vi "FourBarBoth.vi"(10 "Down":dbl, 11 "Up":dbl) -> ()   [LabVIEW 2018]
uses:
  <vilib>/Rock Robotics/WPI/ThirdParty/Phoenix-LabVIEW/Motor Controller/Controls/CTRE_Phoenix_MotorControl_ControlMode.ctl
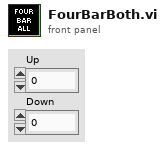
[diagram p1: front panel]
types:
  T1 = typedef "WPI_DigitalInputDevRef.ctl" = cluster{"DevStatus":errorcluster, "DIO Channel":T2}
  T2 = typedef "FPGA_DIOChannel.ctl" = enum8{"DIO 0", "DIO 1", "DIO 2", "DIO 3", "DIO 4", "DIO 5", "DIO 6", "DIO 7", "DIO 8", "DIO 9", "DIO MXP 0", "DIO MXP 1", "DIO MXP 2", "DIO MXP 3", "DIO MXP 4", "DIO MXP 5", "DIO MXP 6", "DIO MXP 7", "DIO MXP 8", "DIO MXP 9", "DIO MXP 10", "DIO MXP 11", "DIO MXP 12", "DIO MXP 13", "DIO MXP 14", "DIO MXP 15", "SPI Port CS1", "SPI Port CS2", "SPI Port CS3", "SPI Port MISO", "SPI Port MOSI", "Invalid"}
  T3 = typedef "CTRE_Phoenix_MotorControl_ControlMode.ctl" = u16
  T4 = typedef "WPI_MotorControlDeviceRef.ctl" = cluster{"DeviceStatus":errorcluster, "Type":T5, "PWM":cluster{"PWM Channel":T6, "DeadBand":T7}, "CAN":cluster{"Device Number":u8, "SetOutput VI Ref":variant, "GetOutput VI Ref":variant, "Enable VI Ref":variant, "Disable VI Ref":variant, "Data":variant}, "Invert":bool, "DIO PWM":cluster{"PWM \"Enable\" Channel":T6, "DIOChannel":T2, "PWM Rate":dbl}}
  T5 = typedef "WPI_MotorControlType.ctl" = enum16{"PWM", "CAN", "DIO PWM"}
  T6 = typedef "FPGA_DIOPWMChannel.ctl" = enum8{"PWM 0", "PWM 1", "PWM 2", "PWM 3", "PWM 4", "PWM 5", "PWM 6", "PWM 7", "PWM 8", "PWM 9", "PWM MXP 0", "PWM MXP 1", "PWM MXP 2", "PWM MXP 3", "PWM MXP 4", "PWM MXP 5", "PWM MXP 6", "PWM MXP 7", "PWM MXP 8", "PWM MXP 9", "Invalid"}
  T7 = typedef "WPI_PWMDeadband.ctl" = cluster{"Name":string, "maxPositivePwm":i32, "minPositivePwm":i32, "centerPwm":i32, "maxNegativePwm":i32, "minNegativePwm":i32, "angularRange":u16}
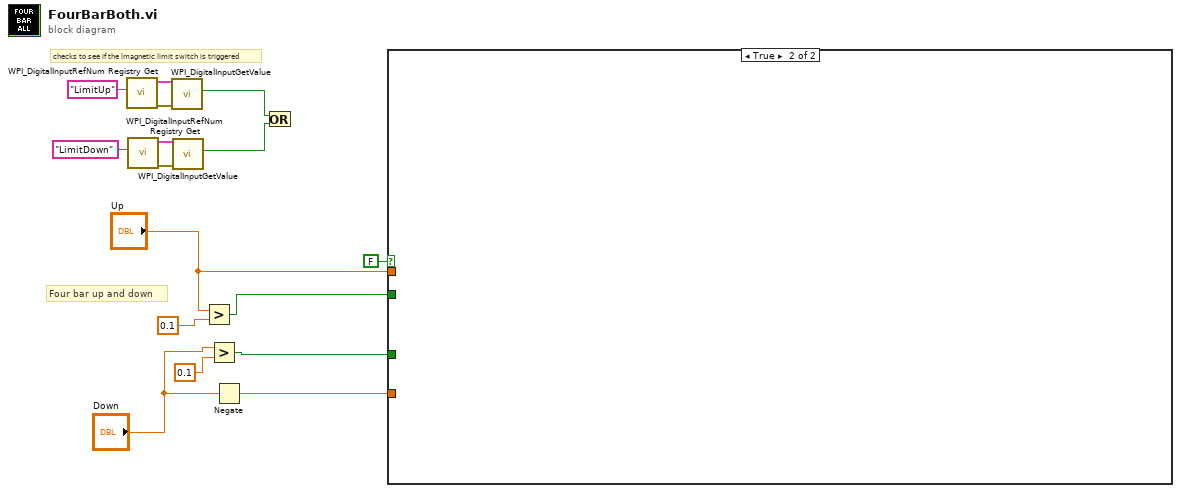
[diagram p0: block diagram]
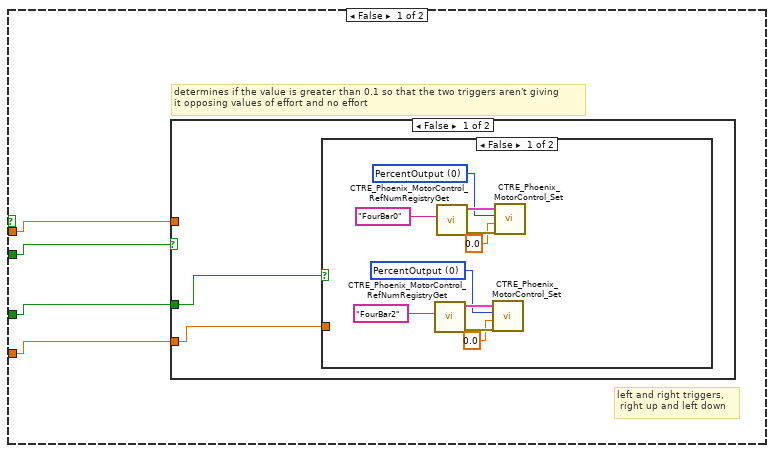
[diagram p2: hidden frame]
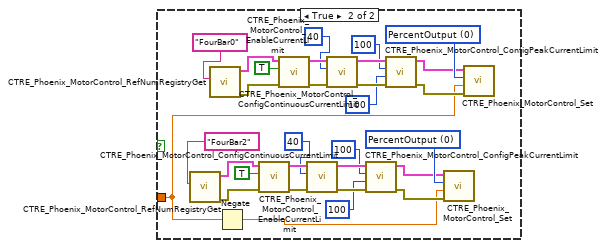
[diagram p3: hidden frame]
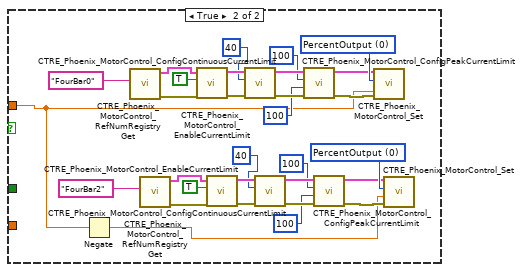
[diagram p4: hidden frame]
diagram:
  # "checks to see if the lmagnetic limit switch is triggered"
  # "Four bar up and down"
  n1 = call <vilib>:"WPI_DigitalInputRefNum Registry Get.vi"("refnum name"="LimitUp") -> ("error out"=w9:errorcluster, "DigitalInputDevRef"=w8:T1)  [unwired: 9 in]
  n2 = call <vilib>:"WPI_DigitalInputRefNum Registry Get.vi"("refnum name"="LimitDown") -> ("error out"=w6:errorcluster, "DigitalInputDevRef"=w5:T1)  [unwired: 9 in]
  n3 = call <vilib>:"WPI_DigitalInputGetValue.vi"("error in (no error)"=w9, "DigitalInputDevRef"=w8) -> ("Value"=w2:bool)  [unwired: 7 in, 2 out]
  n4 = call <vilib>:"WPI_DigitalInputGetValue.vi"("error in (no error)"=w6, "DigitalInputDevRef"=w5) -> ("Value"=w3:bool)  [unwired: 7 in, 2 out]
  n5 = Greater?(x="Up", y=0.1) -> (0:w15:bool)
  n6 = Greater?(x="Down", y=0.1) -> (0:w12:bool)
  n7 = Negate(x="Down") -> (-x=w14:dbl)
  n8 = Or(x=w2, y=w3) -> ()  [unwired: 1 out]
  n9 = case shown="True" FALSE {
    tunnel: w15 -> [w18 _]
    tunnel: w14 -> [w20 _]
    tunnel: w12 -> [w19 _]
    tunnel: "Up" -> [w17 _]
    frame False {
      # "left and right triggers,\n right up and left down"
      # "determines if the value is greater than 0.1 so that the two triggers aren't giving\nit opposing values of effort and no effort"
      n10 = case shown="False" w18 {
        tunnel: w17 -> [_ w64]
        tunnel: w19 -> [w22 _]
        tunnel: w20 -> [w21 _]
        frame False {
          n11 = case shown="False" w22 {
            tunnel: w21 -> [_ w34]
            frame False {
              w24 = T3 0 items=["PercentOutput"=0, "Position"=1, "Velocity"=2, "Current"=3, "Follower"=5, "MotionProfile"=6, "MotionMagic"=7, "MotionMagicArc"=8, "MotionProfileArc"=10, "Disabled"=15] ("Control Mode")
              w29 = T3 0 items=["PercentOutput"=0, "Position"=1, "Velocity"=2, "Current"=3, "Follower"=5, "MotionProfile"=6, "MotionMagic"=7, "MotionMagicArc"=8, "MotionProfileArc"=10, "Disabled"=15] ("Control Mode")
              n12 = call <vilib>:"CTRE_Phoenix_MotorControl_RefNumRegistryGet.vi"("refnum name"="FourBar2") -> ("error out"=w27:errorcluster, "PhoenixMotorControlDevRef"=w26:T4)  [unwired: 9 in]
              n13 = call <vilib>:"CTRE_Phoenix_MotorControl_RefNumRegistryGet.vi"("refnum name"="FourBar0") -> ("error out"=w32:errorcluster, "PhoenixMotorControlDevRef"=w31:T4)  [unwired: 9 in]
              n14 = call <vilib>:"CTRE_Phoenix_MotorControl_Set.vi"("error in (no error)"=w27, "Output"=0.0, "Control Mode"=w24, "PhoenixMotorControlDevRef"=w26) -> ()  [unwired: 6 in, 2 out]
              n15 = call <vilib>:"CTRE_Phoenix_MotorControl_Set.vi"("error in (no error)"=w32, "Output"=0.0, "Control Mode"=w29, "PhoenixMotorControlDevRef"=w31) -> ()  [unwired: 6 in, 2 out]
            }
            frame True {
              w48 = T3 0 items=["PercentOutput"=0, "Position"=1, "Velocity"=2, "Current"=3, "Follower"=5, "MotionProfile"=6, "MotionMagic"=7, "MotionMagicArc"=8, "MotionProfileArc"=10, "Disabled"=15] ("Control Mode")
              w61 = T3 0 items=["PercentOutput"=0, "Position"=1, "Velocity"=2, "Current"=3, "Follower"=5, "MotionProfile"=6, "MotionMagic"=7, "MotionMagicArc"=8, "MotionProfileArc"=10, "Disabled"=15] ("Control Mode")
              n16 = call <vilib>:"CTRE_Phoenix_MotorControl_RefNumRegistryGet.vi"("refnum name"="FourBar2") -> ("error out"=w51:errorcluster, "PhoenixMotorControlDevRef"=w50:T4)  [unwired: 9 in]
              n17 = call <vilib>:"CTRE_Phoenix_MotorControl_RefNumRegistryGet.vi"("refnum name"="FourBar0") -> ("error out"=w39:errorcluster, "PhoenixMotorControlDevRef"=w38:T4)  [unwired: 9 in]
              n18 = Negate(x=w34) -> (-x=w33:dbl)
              n19 = call <vilib>:"CTRE_Phoenix_MotorControl_EnableCurrentLimit.vi"("error in (no error)"=w51, "Enable Current Limit?"=TRUE, "PhoenixMotorControlDevRef"=w50) -> ("error out"=w59:errorcluster, "PhoenixMotorControlDevRef"=w58:T4)  [unwired: 7 in]
              n20 = call <vilib>:"CTRE_Phoenix_MotorControl_EnableCurrentLimit.vi"("error in (no error)"=w39, "Enable Current Limit?"=TRUE, "PhoenixMotorControlDevRef"=w38) -> ("error out"=w46:errorcluster, "PhoenixMotorControlDevRef"=w45:T4)  [unwired: 7 in]
              n21 = call <vilib>:"CTRE_Phoenix_MotorControl_ConfigContinuousCurrentLimit.vi"("error in (no error)"=w59, "Continuous Current Limit (Amps)"=40, "PhoenixMotorControlDevRef"=w58) -> ("error out"=w56:errorcluster, "PhoenixMotorControlDevRef"=w57:T4)  [unwired: 7 in]
              n22 = call <vilib>:"CTRE_Phoenix_MotorControl_ConfigContinuousCurrentLimit.vi"("error in (no error)"=w46, "Continuous Current Limit (Amps)"=40, "PhoenixMotorControlDevRef"=w45) -> ("error out"=w43:errorcluster, "PhoenixMotorControlDevRef"=w44:T4)  [unwired: 7 in]
              n23 = call <vilib>:"CTRE_Phoenix_MotorControl_ConfigPeakCurrentLimit.vi"("error in (no error)"=w56, "Peak Current Maximum Duration (ms)"=100, "Peak Current (Amps)"=100, "PhoenixMotorControlDevRef"=w57) -> ("error out"=w52:errorcluster, "PhoenixMotorControlDevRef"=w53:T4)  [unwired: 6 in]
              n24 = call <vilib>:"CTRE_Phoenix_MotorControl_ConfigPeakCurrentLimit.vi"("error in (no error)"=w43, "Peak Current Maximum Duration (ms)"=100, "Peak Current (Amps)"=100, "PhoenixMotorControlDevRef"=w44) -> ("error out"=w40:errorcluster, "PhoenixMotorControlDevRef"=w41:T4)  [unwired: 6 in]
              n25 = call <vilib>:"CTRE_Phoenix_MotorControl_Set.vi"("error in (no error)"=w52, "Output"=w33, "Control Mode"=w61, "PhoenixMotorControlDevRef"=w53) -> ()  [unwired: 6 in, 2 out]
              n26 = call <vilib>:"CTRE_Phoenix_MotorControl_Set.vi"("error in (no error)"=w40, "Output"=w34, "Control Mode"=w48, "PhoenixMotorControlDevRef"=w41) -> ()  [unwired: 6 in, 2 out]
            }
          }
        }
        frame True {
          w78 = T3 0 items=["PercentOutput"=0, "Position"=1, "Velocity"=2, "Current"=3, "Follower"=5, "MotionProfile"=6, "MotionMagic"=7, "MotionMagicArc"=8, "MotionProfileArc"=10, "Disabled"=15] ("Control Mode")
          w92 = T3 0 items=["PercentOutput"=0, "Position"=1, "Velocity"=2, "Current"=3, "Follower"=5, "MotionProfile"=6, "MotionMagic"=7, "MotionMagicArc"=8, "MotionProfileArc"=10, "Disabled"=15] ("Control Mode")
          n27 = Negate(x=w64) -> (-x=w63:dbl)
          n28 = call <vilib>:"CTRE_Phoenix_MotorControl_RefNumRegistryGet.vi"("refnum name"="FourBar0") -> ("error out"=w83:errorcluster, "PhoenixMotorControlDevRef"=w82:T4)  [unwired: 9 in]
          n29 = call <vilib>:"CTRE_Phoenix_MotorControl_RefNumRegistryGet.vi"("refnum name"="FourBar2") -> ("error out"=w69:errorcluster, "PhoenixMotorControlDevRef"=w68:T4)  [unwired: 9 in]
          n30 = call <vilib>:"CTRE_Phoenix_MotorControl_EnableCurrentLimit.vi"("error in (no error)"=w83, "Enable Current Limit?"=TRUE, "PhoenixMotorControlDevRef"=w82) -> ("error out"=w89:errorcluster, "PhoenixMotorControlDevRef"=w88:T4)  [unwired: 7 in]
          n31 = call <vilib>:"CTRE_Phoenix_MotorControl_EnableCurrentLimit.vi"("error in (no error)"=w69, "Enable Current Limit?"=TRUE, "PhoenixMotorControlDevRef"=w68) -> ("error out"=w75:errorcluster, "PhoenixMotorControlDevRef"=w74:T4)  [unwired: 7 in]
          n32 = call <vilib>:"CTRE_Phoenix_MotorControl_ConfigContinuousCurrentLimit.vi"("error in (no error)"=w89, "Continuous Current Limit (Amps)"=40, "PhoenixMotorControlDevRef"=w88) -> ("error out"=w86:errorcluster, "PhoenixMotorControlDevRef"=w87:T4)  [unwired: 7 in]
          n33 = call <vilib>:"CTRE_Phoenix_MotorControl_ConfigContinuousCurrentLimit.vi"("error in (no error)"=w75, "Continuous Current Limit (Amps)"=40, "PhoenixMotorControlDevRef"=w74) -> ("error out"=w72:errorcluster, "PhoenixMotorControlDevRef"=w73:T4)  [unwired: 7 in]
          n34 = call <vilib>:"CTRE_Phoenix_MotorControl_ConfigPeakCurrentLimit.vi"("error in (no error)"=w86, "Peak Current Maximum Duration (ms)"=100, "Peak Current (Amps)"=100, "PhoenixMotorControlDevRef"=w87) -> ("error out"=w80:errorcluster, "PhoenixMotorControlDevRef"=w81:T4)  [unwired: 6 in]
          n35 = call <vilib>:"CTRE_Phoenix_MotorControl_ConfigPeakCurrentLimit.vi"("error in (no error)"=w72, "Peak Current Maximum Duration (ms)"=100, "Peak Current (Amps)"=100, "PhoenixMotorControlDevRef"=w73) -> ("error out"=w66:errorcluster, "PhoenixMotorControlDevRef"=w67:T4)  [unwired: 6 in]
          n36 = call <vilib>:"CTRE_Phoenix_MotorControl_Set.vi"("error in (no error)"=w80, "Output"=w64, "Control Mode"=w92, "PhoenixMotorControlDevRef"=w81) -> ()  [unwired: 6 in, 2 out]
          n37 = call <vilib>:"CTRE_Phoenix_MotorControl_Set.vi"("error in (no error)"=w66, "Output"=w63, "Control Mode"=w78, "PhoenixMotorControlDevRef"=w67) -> ()  [unwired: 6 in, 2 out]
        }
      }
    }
    frame True {
    }
  }
